vi "Serial Reaction Time Task Controller.vi"() -> ()   [LabVIEW 2016]
uses:
  <vilib>/LabVIEW Interface for Arduino/Type Defs/Board Type.ctl
  <vilib>/Utility/file.llb/Read Delimited Spreadsheet (DBL).vi
  <vilib>/Utility/file.llb/Write Delimited Spreadsheet (DBL).vi
  <vilib>/Utility/file.llb/Write To Spreadsheet File (DBL).vi
  <vilib>/LabVIEW Interface for Arduino/LabVIEW Interface for Arduino.lvlib
panel:
  in  "Debug Mode":bool
  in  "Load Last":bool
  in  "Timeout (sec)":dbl min=0.0 max=1000.0 step=1.0
  in  "Test Mode":bool
  in  "Test Chamber":i32=1 min=1 max=9 step=1
  out "Array":dbl[][](array[numeric])
  in  "Tone":bool
  in  "# of Pellet":i32 max=1000 step=1
  in  "LH (sec)":dbl min=0.0 max=1000.0 step=1.0
  in  "LED On (sec)":dbl min=0.0 max=1000.0 step=1.0
  in  "ITI (sec)":dbl min=0.0 max=1000.0 step=1.0
  in  "# of total Trial":i32 min=0 max=1000 step=1
  in  "Stepper Step":i32 min=0 step=1
  out "ITI":bool
  out "Hole 9":bool
  out "Hole 8":bool
  out "Hole 7":bool
  out "Hole 6":bool
  out "Hole  6":bool
  out "Hole  7":bool
  out "Hole  8":bool
  out "Hole  9":bool
  out "ITI Remaining":dbl format="%<%M:%S>t"
  out "LH Remaining":dbl(slide) scale=0.0..1.0
  out "Experiment Running":bool
  out "Hole 5":bool
  out "Hole 4":bool
  out "Hole 3":bool
  out "Hole 2":bool
  out "Hole 1":bool
  out "Elapsed Time":dbl format="%<%M:%S>t"
  out "Current Trial":dbl
  out "RT (ms)":dbl
  out "Hole  1":bool
  out "Hole  2":bool
  out "Hole  3":bool
  out "Hole  4":bool
  out "Hole  5":bool
  out "Wrong":bool
  out "Correct":bool
  in  "Choice Mode":string(combo)
  out "Detector 2":i32
  out "LED 2":i32
  in  "Set":bool
  in  "Detector Pin":i32=40
  in  "LED Pin":i32=22
  in  "Path":path
  in  "Start":bool
  # "Indicator LED"
  # "Reaction Hole"
  # "to"
  # "to"
  # "# of Trial"
  # "Indicator"
  # "Reaction"
  # "Correct?"
  # "PR?"
  # "# of PMR"
  # "RT(ms)"
  # "Serial Reaction Time Task Controller\nVer 1.0"
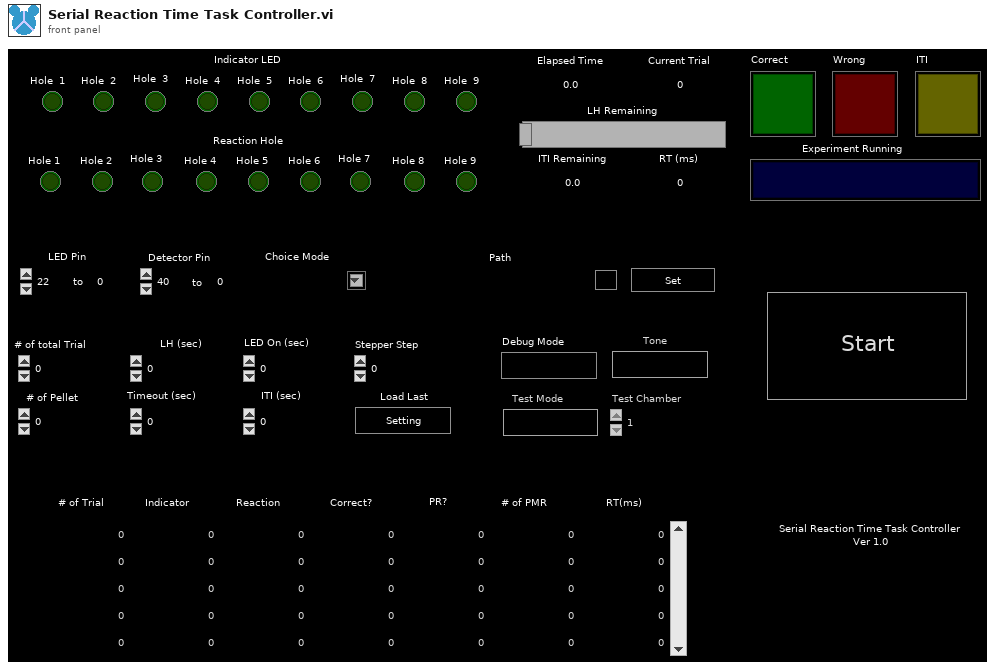
[diagram p1: front panel]
types:
  T1 = typedef "LabVIEW Interface for Arduino.lvlib/Board Type.ctl" = enum16{"Uno", "Dimuelanove w/Atmega 328", "Mega 2560"}
  T2 = enum8{"Enabled", "Disabled", "Disabled and Grayed Out"}
  T3 = typedef "LabVIEW Interface for Arduino.lvlib/Arduino Resource.ctl" = cluster{"VISA resource":refnum<visa-resource-name>, "Board Type":T1, "Connection Type":enum8{"USB / Serial"}, "Bytes Per Packet (15)":u8}
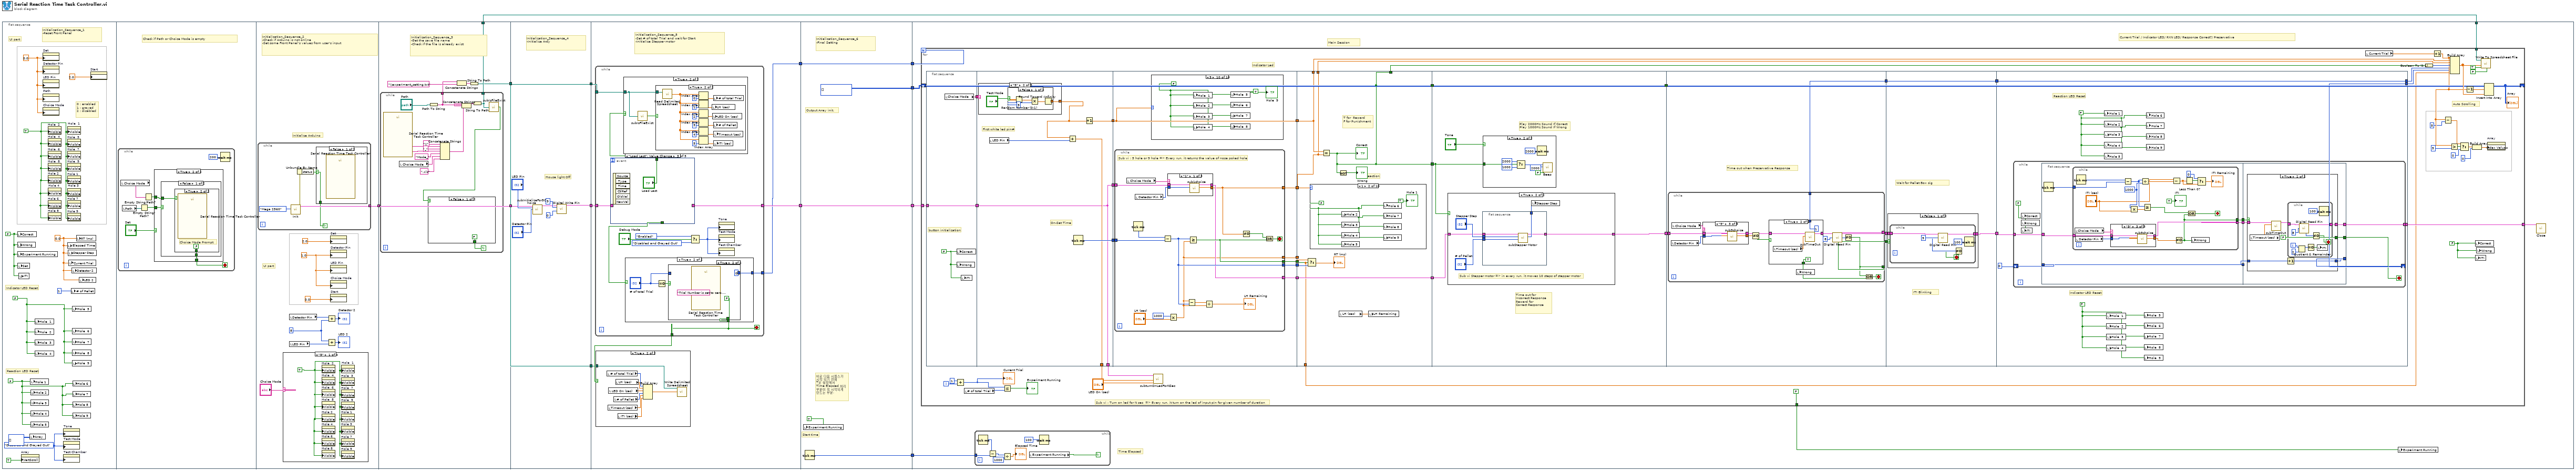
[diagram p0: block diagram]
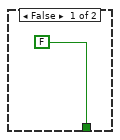
[diagram p2: hidden frame]
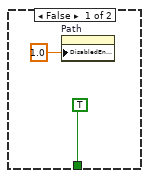
[diagram p3: hidden frame]
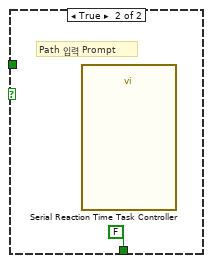
[diagram p4: hidden frame]
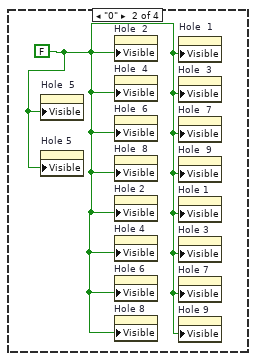
[diagram p5: hidden frame]
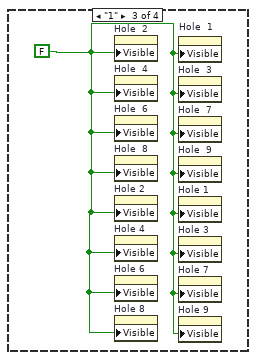
[diagram p6: hidden frame]
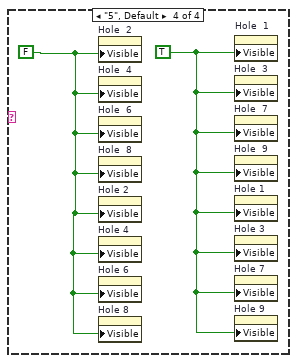
[diagram p7: hidden frame]
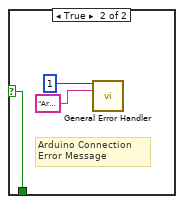
[diagram p8: hidden frame]
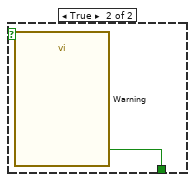
[diagram p9: hidden frame]
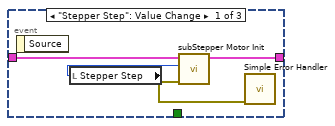
[diagram p11: hidden frame]
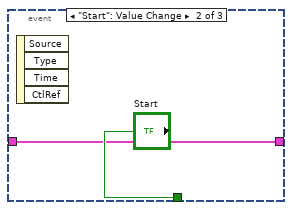
[diagram p12: hidden frame]
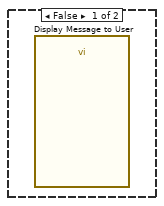
[diagram p14: hidden frame]
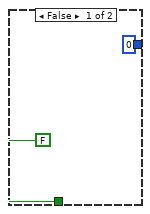
[diagram p15: hidden frame]
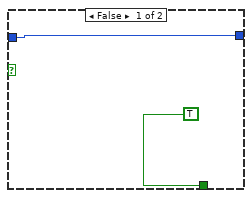
[diagram p16: hidden frame]
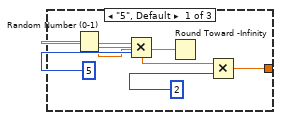
[diagram p17: hidden frame]
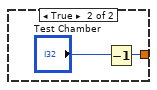
[diagram p18: hidden frame]
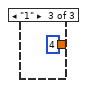
[diagram p19: hidden frame]
diagram:
  n1 = flat-sequence {
    tunnel: [w51] -> w6
    tunnel: [w71] -> w7
    tunnel: w6 -> [w71]
    tunnel: [w70] -> w4
    tunnel: [w67] -> w3
    tunnel: [w88] -> w9
    tunnel: w7 -> [w93]
    tunnel: w3 -> [w92]
    tunnel: [w92] -> w2
    tunnel: [w92] -> w1
    tunnel: [w101] -> w11
    tunnel: [w99] -> w10
    tunnel: w9 -> [w100]
    tunnel: w2 -> [w97]
    tunnel: w1 -> [w96]
    tunnel: [w154] -> w13
    tunnel: [w158] -> w12
    tunnel: w11 -> [w154]
    tunnel: w10 -> [w158]
    tunnel: [w157] -> w8
    tunnel: [i32[][] []] -> w5
    tunnel: w13 -> [w165]
    tunnel: w12 -> [w163]
    tunnel: w8 -> [w162]
    tunnel: w4 -> [w160]
    tunnel: w5 -> [w159]
    frame #0 {
      w14 = T2."Disabled and Grayed Out" ("Disabled")
      w17 = TRUE
      w22 = FALSE
      w23 = FALSE
      w16 = 0.0
      w19 = 0.0
      w18 = FALSE
      # "0 : enabled\n1 : grayed\n2 : disabled"
      # "Initialization_Sequence_1\n-Reset Front Panel"
      # "UI part"
      # "Reaction LED Reset"
      # "Indicator LED Reset"
      n2 = local write "Correct"(w18) -> ()
      n3 = local write "Wrong"(w18) -> ()
      n4 = local write "Experiment Running"(w18) -> ()
      n5 = local write "Set"(w18) -> ()
      n6 = local write "ITI"(w18) -> ()
      n7 = property on="Array" class="Arr (strict)"("VertScroll"=TRUE) -> ()  [unwired: 2 in, 2 out]
      n8 = local write "Array"(i32[][] []) -> ()
      n9 = local write "Hole 1"(w22) -> ()
      n10 = local write "Hole 2"(w22) -> ()
      n11 = local write "Hole 3"(w22) -> ()
      n12 = local write "Hole 4"(w22) -> ()
      n13 = local write "Hole 5"(w22) -> ()
      n14 = local write "Hole  1"(w23) -> ()
      n15 = local write "Hole  2"(w23) -> ()
      n16 = local write "Hole  3"(w23) -> ()
      n17 = local write "Hole  4"(w23) -> ()
      n18 = property on="Set" class="Bool (strict)"("DisabledEnum"=w16) -> ()  [unwired: 2 in, 2 out]
      n19 = property on="Detector Pin" class="DigNum (strict)"("DisabledEnum"=w16) -> ()  [unwired: 2 in, 2 out]
      n20 = property on="LED Pin" class="DigNum (strict)"("DisabledEnum"=w16) -> ()  [unwired: 2 in, 2 out]
      n21 = property on="Path" class="Path"("DisabledEnum"=w16) -> ()  [unwired: 2 in, 2 out]
      n22 = property on="Choice Mode" class="CmbBox"("DisabledEnum"=w16) -> ()  [unwired: 2 in, 2 out]
      n23 = property on="Hole  2" class="Bool (strict)"("Visible"=w17) -> ()  [unwired: 2 in, 2 out]
      n24 = property on="Hole  4" class="Bool (strict)"("Visible"=w17) -> ()  [unwired: 2 in, 2 out]
      n25 = property on="Hole  6" class="Bool (strict)"("Visible"=w17) -> ()  [unwired: 2 in, 2 out]
      n26 = property on="Hole  8" class="Bool (strict)"("Visible"=w17) -> ()  [unwired: 2 in, 2 out]
      n27 = property on="Hole 2" class="Bool (strict)"("Visible"=w17) -> ()  [unwired: 2 in, 2 out]
      n28 = property on="Hole 4" class="Bool (strict)"("Visible"=w17) -> ()  [unwired: 2 in, 2 out]
      n29 = property on="Hole 6" class="Bool (strict)"("Visible"=w17) -> ()  [unwired: 2 in, 2 out]
      n30 = property on="Hole 8" class="Bool (strict)"("Visible"=w17) -> ()  [unwired: 2 in, 2 out]
      n31 = property on="Tone" class="Bool (strict)"("DisabledEnum"=w14) -> ()  [unwired: 2 in, 2 out]
      n32 = property on="Test Mode" class="Bool (strict)"("DisabledEnum"=w14) -> ()  [unwired: 2 in, 2 out]
      n33 = property on="Test Chamber" class="DigNum (strict)"("DisabledEnum"=w14) -> ()  [unwired: 2 in, 2 out]
      n34 = local write "Elapsed Time"(w19) -> ()
      n35 = property on="Hole  1" class="Bool (strict)"("Visible"=w17) -> ()  [unwired: 2 in, 2 out]
      n36 = property on="Hole  3" class="Bool (strict)"("Visible"=w17) -> ()  [unwired: 2 in, 2 out]
      n37 = property on="Hole  7" class="Bool (strict)"("Visible"=w17) -> ()  [unwired: 2 in, 2 out]
      n38 = property on="Hole  9" class="Bool (strict)"("Visible"=w17) -> ()  [unwired: 2 in, 2 out]
      n39 = property on="Hole 1" class="Bool (strict)"("Visible"=w17) -> ()  [unwired: 2 in, 2 out]
      n40 = property on="Hole 3" class="Bool (strict)"("Visible"=w17) -> ()  [unwired: 2 in, 2 out]
      n41 = property on="Hole 7" class="Bool (strict)"("Visible"=w17) -> ()  [unwired: 2 in, 2 out]
      n42 = property on="Hole 9" class="Bool (strict)"("Visible"=w17) -> ()  [unwired: 2 in, 2 out]
      n43 = local write "Stepper Step"(w19) -> ()
      n44 = local write "Current Trial"(w19) -> ()
      n45 = local write "# of Pellet"(1) -> ()
      n46 = local write "Detector 2"(w19) -> ()
      n47 = local write "Hole  5"(w23) -> ()
      n48 = local write "Hole  6"(w23) -> ()
      n49 = local write "Hole  7"(w23) -> ()
      n50 = local write "Hole  8"(w23) -> ()
      n51 = local write "Hole  9"(w23) -> ()
      n52 = local write "Hole 6"(w22) -> ()
      n53 = local write "Hole 7"(w22) -> ()
      n54 = local write "Hole 8"(w22) -> ()
      n55 = local write "Hole 9"(w22) -> ()
      n56 = local write "RT (ms)"(w19) -> ()
      n57 = local write "LED 2"(w19) -> ()
      n58 = property on="Start" class="Bool (strict)"("DisabledEnum"=2.0) -> ()  [unwired: 2 in, 2 out]
    }
    frame #1 {
      # "Check if Path or Choice Mode is empty"
      n59 = while {
        stop <- w31 stop-if-true
        n60 = local read "Choice Mode"() -> (w26:string)
        n61 = local read "Path"() -> (w29:path)
        n62 = Empty String/Path?(string/path=w29) -> (empty?=w30:bool)
        n63 = Empty String/Path?(string/path=w26) -> (empty?=w27:bool)
        n64 = case shown="True" "Set" {
          tunnel: [FALSE w35] -> w31
          tunnel: w30 -> [_ w34]
          tunnel: w27 -> [_ w33]
          frame False {
          }
          frame True {
            n65 = case shown="False" w34 {
              tunnel: [w36 FALSE] -> w35
              tunnel: w33 -> [w37 _]
              frame False {
                n66 = case shown="True" w37 {
                  tunnel: [TRUE FALSE] -> w36
                  frame False {
                    n67 = property on="Path" class="Path"("DisabledEnum"=1.0) -> ()  [unwired: 2 in, 2 out]
                  }
                  frame True {
                    # "Choice Mode Prompt"
                    n68 = call "Serial Reaction Time Task Controller"() -> ()  [unwired: 10 in, 2 out]
                  }
                }
              }
              frame True {
                # "Path 입력 Prompt"
                n69 = call "Serial Reaction Time Task Controller"() -> ()  [unwired: 10 in, 2 out]
              }
            }
          }
        }
        n70 = Wait (ms)(milliseconds to wait=u32 200) -> ()  [unwired: 1 out]
      }
    }
    frame #2 {
      w46 = 8
      w47 = 1.0
      # "Initialize Arduino"
      # "UI part"
      # "Initialization_Sequence_2\n-Check if Arduino is not online\n-Set some Front Panel's values from user's input"
      n71 = while {
        tunnel: [w60] -> w51
        stop <- w57 continue-if-true
        n72 = call <vilib>:"Init.vi"("Board Type (Uno)"=Board_Type."Mega 2560") -> ("Arduino Resource"=w60:T3, "error out"=w59:errorcluster)  [unwired: 17 in]
        n73 = Unbundle By Name(w59) -> ("status"=w58:bool)
        n74 = case shown="False" w58 {
          selector: w58 -> [w62 w63]
          tunnel: [w62 w63] -> w57
          frame False {
            n75 = call "Serial Reaction TIme Task Controller"() -> ()  [unwired: 10 in, 2 out]
          }
          frame True {
            # "Arduino Connection\nError Message"
            n76 = call <vilib>:"General Error Handler.vi"("[error code] (0)"=1, "[error source] (\" \")"="Arduino Connection Error. Check USB port or plug USB port out and in again." ("[error source] (\" \")")) -> ()  [unwired: 9 in, 5 out]
          }
        }
      }
      n77 = case shown="\"9\"" "Choice Mode" {
        frame "9" {
          w52 = TRUE
          n78 = property on="Hole  2" class="Bool (strict)"("Visible"=w52) -> ()  [unwired: 2 in, 2 out]
          n79 = property on="Hole  4" class="Bool (strict)"("Visible"=w52) -> ()  [unwired: 2 in, 2 out]
          n80 = property on="Hole  6" class="Bool (strict)"("Visible"=w52) -> ()  [unwired: 2 in, 2 out]
          n81 = property on="Hole  8" class="Bool (strict)"("Visible"=w52) -> ()  [unwired: 2 in, 2 out]
          n82 = property on="Hole 2" class="Bool (strict)"("Visible"=w52) -> ()  [unwired: 2 in, 2 out]
          n83 = property on="Hole 4" class="Bool (strict)"("Visible"=w52) -> ()  [unwired: 2 in, 2 out]
          n84 = property on="Hole 6" class="Bool (strict)"("Visible"=w52) -> ()  [unwired: 2 in, 2 out]
          n85 = property on="Hole 8" class="Bool (strict)"("Visible"=w52) -> ()  [unwired: 2 in, 2 out]
          n86 = property on="Hole  1" class="Bool (strict)"("Visible"=w52) -> ()  [unwired: 2 in, 2 out]
          n87 = property on="Hole  3" class="Bool (strict)"("Visible"=w52) -> ()  [unwired: 2 in, 2 out]
          n88 = property on="Hole  7" class="Bool (strict)"("Visible"=w52) -> ()  [unwired: 2 in, 2 out]
          n89 = property on="Hole  9" class="Bool (strict)"("Visible"=w52) -> ()  [unwired: 2 in, 2 out]
          n90 = property on="Hole 1" class="Bool (strict)"("Visible"=w52) -> ()  [unwired: 2 in, 2 out]
          n91 = property on="Hole 3" class="Bool (strict)"("Visible"=w52) -> ()  [unwired: 2 in, 2 out]
          n92 = property on="Hole 7" class="Bool (strict)"("Visible"=w52) -> ()  [unwired: 2 in, 2 out]
          n93 = property on="Hole 9" class="Bool (strict)"("Visible"=w52) -> ()  [unwired: 2 in, 2 out]
        }
        frame "0" {
          w53 = FALSE
          n94 = property on="Hole  5" class="Bool (strict)"("Visible"=w53) -> ()  [unwired: 2 in, 2 out]
          n95 = property on="Hole 5" class="Bool (strict)"("Visible"=w53) -> ()  [unwired: 2 in, 2 out]
          n96 = property on="Hole  2" class="Bool (strict)"("Visible"=w53) -> ()  [unwired: 2 in, 2 out]
          n97 = property on="Hole  4" class="Bool (strict)"("Visible"=w53) -> ()  [unwired: 2 in, 2 out]
          n98 = property on="Hole  6" class="Bool (strict)"("Visible"=w53) -> ()  [unwired: 2 in, 2 out]
          n99 = property on="Hole  8" class="Bool (strict)"("Visible"=w53) -> ()  [unwired: 2 in, 2 out]
          n100 = property on="Hole 2" class="Bool (strict)"("Visible"=w53) -> ()  [unwired: 2 in, 2 out]
          n101 = property on="Hole 4" class="Bool (strict)"("Visible"=w53) -> ()  [unwired: 2 in, 2 out]
          n102 = property on="Hole 6" class="Bool (strict)"("Visible"=w53) -> ()  [unwired: 2 in, 2 out]
          n103 = property on="Hole 8" class="Bool (strict)"("Visible"=w53) -> ()  [unwired: 2 in, 2 out]
          n104 = property on="Hole  1" class="Bool (strict)"("Visible"=w53) -> ()  [unwired: 2 in, 2 out]
          n105 = property on="Hole  3" class="Bool (strict)"("Visible"=w53) -> ()  [unwired: 2 in, 2 out]
          n106 = property on="Hole  7" class="Bool (strict)"("Visible"=w53) -> ()  [unwired: 2 in, 2 out]
          n107 = property on="Hole  9" class="Bool (strict)"("Visible"=w53) -> ()  [unwired: 2 in, 2 out]
          n108 = property on="Hole 1" class="Bool (strict)"("Visible"=w53) -> ()  [unwired: 2 in, 2 out]
          n109 = property on="Hole 3" class="Bool (strict)"("Visible"=w53) -> ()  [unwired: 2 in, 2 out]
          n110 = property on="Hole 7" class="Bool (strict)"("Visible"=w53) -> ()  [unwired: 2 in, 2 out]
          n111 = property on="Hole 9" class="Bool (strict)"("Visible"=w53) -> ()  [unwired: 2 in, 2 out]
        }
        frame "1" {
          w54 = FALSE
          n112 = property on="Hole  2" class="Bool (strict)"("Visible"=w54) -> ()  [unwired: 2 in, 2 out]
          n113 = property on="Hole  4" class="Bool (strict)"("Visible"=w54) -> ()  [unwired: 2 in, 2 out]
          n114 = property on="Hole  6" class="Bool (strict)"("Visible"=w54) -> ()  [unwired: 2 in, 2 out]
          n115 = property on="Hole  8" class="Bool (strict)"("Visible"=w54) -> ()  [unwired: 2 in, 2 out]
          n116 = property on="Hole 2" class="Bool (strict)"("Visible"=w54) -> ()  [unwired: 2 in, 2 out]
          n117 = property on="Hole 4" class="Bool (strict)"("Visible"=w54) -> ()  [unwired: 2 in, 2 out]
          n118 = property on="Hole 6" class="Bool (strict)"("Visible"=w54) -> ()  [unwired: 2 in, 2 out]
          n119 = property on="Hole 8" class="Bool (strict)"("Visible"=w54) -> ()  [unwired: 2 in, 2 out]
          n120 = property on="Hole  1" class="Bool (strict)"("Visible"=w54) -> ()  [unwired: 2 in, 2 out]
          n121 = property on="Hole  3" class="Bool (strict)"("Visible"=w54) -> ()  [unwired: 2 in, 2 out]
          n122 = property on="Hole  7" class="Bool (strict)"("Visible"=w54) -> ()  [unwired: 2 in, 2 out]
          n123 = property on="Hole  9" class="Bool (strict)"("Visible"=w54) -> ()  [unwired: 2 in, 2 out]
          n124 = property on="Hole 1" class="Bool (strict)"("Visible"=w54) -> ()  [unwired: 2 in, 2 out]
          n125 = property on="Hole 3" class="Bool (strict)"("Visible"=w54) -> ()  [unwired: 2 in, 2 out]
          n126 = property on="Hole 7" class="Bool (strict)"("Visible"=w54) -> ()  [unwired: 2 in, 2 out]
          n127 = property on="Hole 9" class="Bool (strict)"("Visible"=w54) -> ()  [unwired: 2 in, 2 out]
        }
        frame "5", Default {
          w55 = TRUE
          w56 = FALSE
          n128 = property on="Hole  2" class="Bool (strict)"("Visible"=w56) -> ()  [unwired: 2 in, 2 out]
          n129 = property on="Hole  4" class="Bool (strict)"("Visible"=w56) -> ()  [unwired: 2 in, 2 out]
          n130 = property on="Hole  6" class="Bool (strict)"("Visible"=w56) -> ()  [unwired: 2 in, 2 out]
          n131 = property on="Hole  8" class="Bool (strict)"("Visible"=w56) -> ()  [unwired: 2 in, 2 out]
          n132 = property on="Hole 2" class="Bool (strict)"("Visible"=w56) -> ()  [unwired: 2 in, 2 out]
          n133 = property on="Hole 4" class="Bool (strict)"("Visible"=w56) -> ()  [unwired: 2 in, 2 out]
          n134 = property on="Hole 6" class="Bool (strict)"("Visible"=w56) -> ()  [unwired: 2 in, 2 out]
          n135 = property on="Hole 8" class="Bool (strict)"("Visible"=w56) -> ()  [unwired: 2 in, 2 out]
          n136 = property on="Hole  1" class="Bool (strict)"("Visible"=w55) -> ()  [unwired: 2 in, 2 out]
          n137 = property on="Hole  3" class="Bool (strict)"("Visible"=w55) -> ()  [unwired: 2 in, 2 out]
          n138 = property on="Hole  7" class="Bool (strict)"("Visible"=w55) -> ()  [unwired: 2 in, 2 out]
          n139 = property on="Hole  9" class="Bool (strict)"("Visible"=w55) -> ()  [unwired: 2 in, 2 out]
          n140 = property on="Hole 1" class="Bool (strict)"("Visible"=w55) -> ()  [unwired: 2 in, 2 out]
          n141 = property on="Hole 3" class="Bool (strict)"("Visible"=w55) -> ()  [unwired: 2 in, 2 out]
          n142 = property on="Hole 7" class="Bool (strict)"("Visible"=w55) -> ()  [unwired: 2 in, 2 out]
          n143 = property on="Hole 9" class="Bool (strict)"("Visible"=w55) -> ()  [unwired: 2 in, 2 out]
        }
      }
      n144 = local read "Detector Pin"() -> (w45:i32)
      n145 = local read "LED Pin"() -> (w43:i32)
      n146 = Add(x=w45, y=w46) -> (x+y=→"Detector 2":i32)
      n147 = Add(x=w46, y=w43) -> (x+y=→"LED 2":i32)
      n148 = property on="Set" class="Bool (strict)"("DisabledEnum"=2.0) -> ()  [unwired: 2 in, 2 out]
      n149 = property on="Detector Pin" class="DigNum (strict)"("DisabledEnum"=w47) -> ()  [unwired: 2 in, 2 out]
      n150 = property on="LED Pin" class="DigNum (strict)"("DisabledEnum"=w47) -> ()  [unwired: 2 in, 2 out]
      n151 = property on="Choice Mode" class="CmbBox"("DisabledEnum"=w47) -> ()  [unwired: 2 in, 2 out]
      n152 = property on="Start" class="Bool (strict)"("DisabledEnum"=0.0) -> ()  [unwired: 2 in, 2 out]
    }
    frame #3 {
      # "Initialization_Sequence_3\n-Get the save file name\n-Check if the file is already exist"
      n153 = while {
        tunnel: [w77] -> w70
        tunnel: [w75] -> w66
        stop <- w78 continue-if-true
        n154 = call "Serial Reaction Time Task Controller"() -> ("Subject number"=w84:string, "Experiment name"=w82:string)  [unwired: 16 in, 2 out]
        n155 = local read "Choice Mode"() -> (w72:string)
        n156 = Path To String(path="Path") -> (string=w75:string)
        n157 = Concatenate Strings("\\", w82, "_", w84, "Mode_", w72, ".xls") -> (w80:string)
        n158 = Concatenate Strings(w75, w80) -> (w81:string)
        n159 = String To Path(string=w81) -> (path=w77:path)
        n160 = call "subIsFileExist.vi"("Path"=w77) -> ("isFileExist"=w79:bool)
        n161 = case shown="False" w79 {
          tunnel: [FALSE w87] -> w78
          frame False {
          }
          frame True {
            n162 = call "Warning"() -> ("Change"=w87:bool)  [unwired: 18 in, 1 out]
          }
        }
      }
      n163 = Concatenate Strings(w66, "\\experiment_setting.txt" ("string")) -> (w68:string)
      n164 = String To Path(string=w68) -> (path=w67:path)
    }
    frame #4 {
      # "House light Off"
      # "Initialization_Sequence_4\n-Initialize Ardy"
      n165 = call "subInitializeFor5Choice.vi"("Arduino Resource"=w93, "LED Start Pin"="LED Pin", "Detector Start Pin"="Detector Pin") -> ("Arduino Resource 2"=w89:T3)  [unwired: 11 in, 1 out]
      n166 = call <vilib>:"Digital Write Pin.vi"("Arduino Resource"=w89, "Digital I/O Pin (0)"=9, "Value (0)"=0) -> ("Arduino Resource"=w88:T3)  [unwired: 11 in, 1 out]
    }
    frame #5 {
      # "Initialization_Sequence_5\n-Set # of total Trial and wait for Start\n-Initialize Stepper motor"
      n167 = while {
        tunnel: [w112] -> w101
        tunnel: w100 -> [w113]
        tunnel: [w120] -> w99
        tunnel: [w115] -> w98
        tunnel: w96 -> [w114]
        stop <- w115 stop-if-true
        n168 = event shown="[2] \"Load Last\": Value Change" {
          selector: _ -> [_ _ _]
          dyn-events: _ -> [_ _ _]
          timeout: _ -> [_ _ _]
          tunnel: w113 -> [w124 w125 _]
          tunnel: [w123 w125 _] -> w112
          tunnel: [_ "Start" _] -> w111
          tunnel: [_ _ "Load Last"] -> w110
          event "Stepper Step": Value Change {
            n169 = event-data() -> ()  [unwired: 1 in, 1 out]
            n170 = local read "Stepper Step"() -> (w121:i32)
            n171 = call "subStepper Motor Init.vi"("Numeric"=w121, "Arduino Resource"=w124) -> ("error out"=w122:errorcluster, "Arduino Resource 2"=w123:T3)  [unwired: 8 in]
            n172 = call <vilib>:"Simple Error Handler.vi"("error in (no error)"=w122) -> ()  [unwired: 4 in, 5 out]
          }
          event "Start": Value Change {
            n173 = event-data() -> ()  [unwired: 1 in, 4 out]
          }
          event "Load Last": Value Change {
            n174 = event-data() -> ()  [unwired: 1 in, 6 out]
          }
        }
        n175 = case shown="True" w110 {
          tunnel: w114 -> [_ w129]
          frame False {
          }
          frame True {
            n176 = call "subIsFileExist.vi"("Path"=w129) -> ("isFileExist"=w128:bool)
            n177 = case shown="True" w128 {
              tunnel: w129 -> [_ w131]
              frame False {
                n178 = call "Display Message to User"() -> ()  [unwired: 10 in, 2 out]
              }
              frame True {
                n179 = call-poly <vilib>:"Read Delimited Spreadsheet.vi"("file path (dialog if empty)"=w131) -> ("first row"=w130:dbl[])  [unwired: 9 in, 5 out]
                n180 = Index Array(array=w130, index=0) -> (element=w143:dbl)
                n181 = Index Array(array=w130, index=1) -> (element=w142:dbl)
                n182 = Index Array(array=w130, index=2) -> (element=w141:dbl)
                n183 = Index Array(array=w130, index=3) -> (element=w140:dbl)
                n184 = Index Array(array=w130, index=4) -> (element=w139:dbl)
                n185 = Index Array(array=w130, index=5) -> (element=w138:dbl)
                n186 = local write "LH (sec)"(w142) -> ()
                n187 = local write "LED On (sec)"(w141) -> ()
                n188 = local write "# of total Trial"(w143) -> ()
                n189 = local write "# of Pellet"(w140) -> ()
                n190 = local write "Timeout (sec)"(w139) -> ()
                n191 = local write "ITI (sec)"(w138) -> ()
              }
            }
          }
        }
        n192 = case shown="True" w111 {
          tunnel: [0 ("# of total Trial") w146] -> w120
          tunnel: [FALSE w148] -> w115
          frame False {
          }
          frame True {
            n193 = Equal To 0?(x="# of total Trial") -> (x = 0?=w149:bool)
            n194 = case shown="True" w149 {
              tunnel: [TRUE FALSE] -> w148
              tunnel: "# of total Trial" -> [w151 _]
              tunnel: [w151 0 ("# of total Trial")] -> w146
              frame False {
              }
              frame True {
                (unwired) "Trial Number is set to zero. Please change the value" ("error source (\" \")")
                n195 = call "Serial Reaction Time Task Controller"() -> ()  [unwired: 10 in, 2 out]
              }
            }
          }
        }
        n196 = Select(t=T2."Enabled" ("Disabled"), s="Debug Mode", f=T2."Disabled and Grayed Out" ("Disabled")) -> (s? t:f=w116:T2)
        n197 = property on="Tone" class="Bool (strict)"("DisabledEnum"=w116) -> ()  [unwired: 2 in, 2 out]
        n198 = property on="Test Mode" class="Bool (strict)"("DisabledEnum"=w116) -> ()  [unwired: 2 in, 2 out]
        n199 = property on="Test Chamber" class="DigNum (strict)"("DisabledEnum"=w116) -> ()  [unwired: 2 in, 2 out]
      }
      n200 = case shown="True" w98 {
        tunnel: w97 -> [_ w103]
        frame False {
        }
        frame True {
          n201 = local read "# of total Trial"() -> (w109:i32)
          n202 = local read "Timeout (sec)"() -> (w105:dbl)
          n203 = local read "LED On (sec)"() -> (w107:dbl)
          n204 = local read "# of Pellet"() -> (w106:i32)
          n205 = local read "LH (sec)"() -> (w108:dbl)
          n206 = local read "ITI (sec)"() -> (w104:dbl)
          n207 = Build Array(w109, w108, w107, w106, w105, w104) -> (w102:dbl[])
          n208 = call-poly <vilib>:"Write Delimited Spreadsheet.vi"("file path (dialog if empty)"=w103, "1D data"=w102) -> ()  [unwired: 12 in, 2 out]
        }
      }
    }
    frame #6 {
      # "Output Array init."
      # "Initialization_Sequence_6\n-Final Setting"
      # "바로 다음 시퀀스가\n시작 되기 전에 \nT로 설정해서 \nTime Elapsed 처리\n부분이 꼭 시작되게\n만드는 부분."
      # "Start time"
      n209 = local write "Experiment Running"(TRUE) -> ()
      n210 = Tick Count (ms)() -> (millisecond timer value=w157:u32)
    }
    frame #7 {
      # "Current Trial / Indicator LED/ RXN LED/ Response Correct?/ Preservative"
      # "Time Elapsed"
      # "Main Session"
      n211 = for {
        N: w163 -> [_]
        tunnel: w165 -> [w224]
        tunnel: [w220] -> w164
        tunnel: [FALSE] -> w161
        tunnel: w160 -> [w207]
        shift-right: [w200] -> _
        shift-left: w159 -> [w201]
        i -> [w217]
        w174 = FALSE
        # "Indicator Led"
        # "Auto Scrolling"
        # "Sub vi : Turn on led for N sec  => Every run, it turn on the led of input pin for given number of duration"
        n212 = flat-sequence {
          tunnel: w224 -> [w232]
          tunnel: [w232] -> w223
          tunnel: [w231] -> w208
          tunnel: [w233] -> w229
          tunnel: [w239] -> w228
          tunnel: w223 -> [w237]
          tunnel: [w237] -> w212
          tunnel: [w238] -> w213
          tunnel: [w237] -> w222
          tunnel: w208 -> [w235]
          tunnel: w229 -> [w256]
          tunnel: w228 -> [w262]
          tunnel: [w256] -> w227
          tunnel: [w261] -> w226
          tunnel: [w260] -> w225
          tunnel: w222 -> [w259]
          tunnel: [w258] -> w221
          tunnel: [w257] -> w219
          tunnel: [w255] -> w209
          tunnel: w227 -> [w314]
          tunnel: w226 -> [w309]
          tunnel: w225 -> [w316]
          tunnel: [w318] -> w185
          tunnel: w221 -> [w318]
          tunnel: [w312] -> w184
          tunnel: w219 -> [w315]
          tunnel: [w314] -> w206
          tunnel: [w309] -> w205
          tunnel: [w312] -> w218
          tunnel: w209 -> [w313]
          tunnel: [w312] -> w183
          tunnel: [w311] -> w175
          tunnel: [w341] -> w187
          tunnel: [w340] -> w186
          tunnel: w183 -> [w340]
          tunnel: w184 -> [w338]
          tunnel: w185 -> [w342]
          tunnel: w187 -> [w366]
          tunnel: [w365] -> w181
          tunnel: w186 -> [_]
          tunnel: [w364] -> w179
          tunnel: [w363] -> w177
          tunnel: w181 -> [w403]
          tunnel: [w402] -> w180
          tunnel: w179 -> [w404]
          tunnel: [w404] -> w178
          tunnel: w177 -> [w401]
          tunnel: w180 -> [w417]
          tunnel: [w418] -> w220
          tunnel: w178 -> [w416]
          tunnel: [w416] -> w182
          tunnel: [w414] -> w176
          frame #0 {
            w230 = FALSE
            # "button initialization"
            n213 = local read "Choice Mode"() -> (w231:string)
            n214 = local write "Correct"(w230) -> ()
            n215 = local write "Wrong"(w230) -> ()
            n216 = local write "ITI"(w230) -> ()
          }
          frame #1 {
            # "On-Set Time"
            # "First white led pin#"
            n217 = case shown="\"9\"" w235 {
              tunnel: [w240 w247 4] -> w234
              frame "5", Default {
                n218 = Random Number (0-1)() -> (number: 0 to 1=w244:dbl)
                n219 = Multiply(x=w244, y=5) -> (x*y=w241:dbl)
                n220 = Round Toward -Infinity(1:w241) -> (0:w242:dbl)
                n221 = Multiply(x=w242, y=2) -> (x*y=w240:dbl)
              }
              frame "9" {
                n222 = case shown="False" "Test Mode" {
                  tunnel: [w248 w252] -> w247
                  frame False {
                    n223 = Random Number (0-1)() -> (number: 0 to 1=w251:dbl)
                    n224 = Multiply(x=w251, y=9) -> (x*y=w249:dbl)
                    n225 = Round Toward -Infinity(1:w249) -> (0:w248:dbl)
                  }
                  frame True {
                    n226 = Decrement(x="Test Chamber") -> (x-1=w252:i32)
                  }
                }
              }
              frame "1" {
              }
            }
            n227 = local read "LED Pin"() -> (w236:i32)
            n228 = Add(x=w234, y=w236) -> (x+y=w238:dbl)
            n229 = Tick Count (ms)() -> (millisecond timer value=w239:u32)
            n230 = Increment(x=w234) -> (x+1=w233:dbl)
          }
          frame #2 {
            n231 = while {
              tunnel: w262 -> [w294]
              tunnel: [w287] -> w261
              tunnel: [w291] -> w260
              tunnel: w259 -> [w289]
              tunnel: [w288] -> w258
              tunnel: [w292] -> w257
              tunnel: [w283] -> w255
              stop <- w296 stop-if-true
              # "Sub vi : 5 hole or 9 hole => Every run, it returns the value of nose poked hole"
              n232 = local read "Choice Mode"() -> (w290:string)
              n233 = Tick Count (ms)() -> (millisecond timer value=w293:u32)
              n234 = local read "Detector Pin"() -> (w284:i32)
              n235 = Subtract(x=w293, y=w294) -> (x-y=w291:u32)
              n236 = case shown="\"1\"" w290 {
                tunnel: [w299 w303 w308] -> w288
                tunnel: w289 -> [w300 w304 w306]
                tunnel: [w298 w302 w307] -> w287
                tunnel: w284 -> [w297 w301 w305]
                frame "1" {
                  n237 = call "sub1choice.vi"("Detector Start Pin"=w297, "Arduino Resource"=w300) -> ("Numeric"=w298:dbl, "Arduino Resource 2"=w299:T3)  [unwired: 7 in, 1 out]
                }
                frame "5", Default {
                  n238 = call "sub5choice.vi"("Detector Start Pin"=w301, "Arduino Resource"=w304) -> ("Numeric"=w302:dbl, "Arduino Resource 2"=w303:T3)  [unwired: 7 in, 1 out]
                }
                frame "9" {
                  n239 = call "sub9choice.vi"("Detector Start Pin"=w305, "Arduino Resource"=w306) -> ("Ouput"=w307:dbl, "Arduino Resource 2"=w308:T3)  [unwired: 7 in, 1 out]
                }
              }
              n240 = Multiply(x=1000, y="LH (sec)") -> (x*y=w283:dbl)
              n241 = Subtract(x=w283, y=w291) -> (x-y=w282:dbl)
              n242 = Greater Or Equal?(x=w291, y=w283) -> (x >= y?=w292:bool)
              n243 = Divide(x=w282, y=w283) -> (x/y=→"LH Remaining":dbl)
              n244 = Not Equal To 0?(x=w287) -> (x != 0?=w295:bool)
              n245 = Or(x=w295, y=w292) -> (x .or. y?=w296:bool)
            }
            n246 = case shown="9" w256 {
              frame 0, Default {
              }
              frame 1 {
                w263 = FALSE
                n247 = local write "Hole  2"(w263) -> ()
                n248 = local write "Hole  3"(w263) -> ()
                n249 = local write "Hole  4"(w263) -> ()
                n250 = local write "Hole  5"(w263) -> ()
                n251 = local write "Hole  6"(w263) -> ()
                n252 = local write "Hole  7"(w263) -> ()
                n253 = local write "Hole  8"(w263) -> ()
                n254 = local write "Hole  9"(w263) -> ()
                "Hole  1" <- TRUE
              }
              frame 2 {
                w265 = FALSE
                n255 = local write "Hole  1"(w265) -> ()
                n256 = local write "Hole  3"(w265) -> ()
                n257 = local write "Hole  4"(w265) -> ()
                n258 = local write "Hole  5"(w265) -> ()
                n259 = local write "Hole  6"(w265) -> ()
                n260 = local write "Hole  7"(w265) -> ()
                n261 = local write "Hole  8"(w265) -> ()
                n262 = local write "Hole  9"(w265) -> ()
                "Hole  2" <- TRUE
              }
              frame 3 {
                w267 = FALSE
                n263 = local write "Hole  1"(w267) -> ()
                n264 = local write "Hole  2"(w267) -> ()
                n265 = local write "Hole  4"(w267) -> ()
                n266 = local write "Hole  5"(w267) -> ()
                n267 = local write "Hole  6"(w267) -> ()
                n268 = local write "Hole  7"(w267) -> ()
                n269 = local write "Hole  8"(w267) -> ()
                n270 = local write "Hole  9"(w267) -> ()
                "Hole  3" <- TRUE
              }
              frame 4 {
                w269 = FALSE
                n271 = local write "Hole  1"(w269) -> ()
                n272 = local write "Hole  2"(w269) -> ()
                n273 = local write "Hole  3"(w269) -> ()
                n274 = local write "Hole  5"(w269) -> ()
                n275 = local write "Hole  6"(w269) -> ()
                n276 = local write "Hole  7"(w269) -> ()
                n277 = local write "Hole  8"(w269) -> ()
                n278 = local write "Hole  9"(w269) -> ()
                "Hole  4" <- TRUE
              }
              frame 5 {
                w271 = FALSE
                n279 = local write "Hole  1"(w271) -> ()
                n280 = local write "Hole  2"(w271) -> ()
                n281 = local write "Hole  3"(w271) -> ()
                n282 = local write "Hole  4"(w271) -> ()
                n283 = local write "Hole  6"(w271) -> ()
                n284 = local write "Hole  7"(w271) -> ()
                n285 = local write "Hole  8"(w271) -> ()
                n286 = local write "Hole  9"(w271) -> ()
                "Hole  5" <- TRUE
              }
              frame 6 {
                w274 = FALSE
                n287 = local write "Hole  1"(w274) -> ()
                n288 = local write "Hole  2"(w274) -> ()
                n289 = local write "Hole  3"(w274) -> ()
                n290 = local write "Hole  4"(w274) -> ()
                n291 = local write "Hole  5"(w274) -> ()
                n292 = local write "Hole  7"(w274) -> ()
                n293 = local write "Hole  8"(w274) -> ()
                n294 = local write "Hole  9"(w274) -> ()
                "Hole  6" <- TRUE
              }
              frame 7 {
                w276 = FALSE
                n295 = local write "Hole  1"(w276) -> ()
                n296 = local write "Hole  2"(w276) -> ()
                n297 = local write "Hole  3"(w276) -> ()
                n298 = local write "Hole  4"(w276) -> ()
                n299 = local write "Hole  5"(w276) -> ()
                n300 = local write "Hole  6"(w276) -> ()
                n301 = local write "Hole  8"(w276) -> ()
                n302 = local write "Hole  9"(w276) -> ()
                "Hole  7" <- TRUE
              }
              frame 8 {
                w278 = FALSE
                n303 = local write "Hole  1"(w278) -> ()
                n304 = local write "Hole  2"(w278) -> ()
                n305 = local write "Hole  3"(w278) -> ()
                n306 = local write "Hole  4"(w278) -> ()
                n307 = local write "Hole  5"(w278) -> ()
                n308 = local write "Hole  6"(w278) -> ()
                n309 = local write "Hole  7"(w278) -> ()
                n310 = local write "Hole  9"(w278) -> ()
                "Hole  8" <- TRUE
              }
              frame 9 {
                w280 = FALSE
                n311 = local write "Hole  1"(w280) -> ()
                n312 = local write "Hole  2"(w280) -> ()
                n313 = local write "Hole  3"(w280) -> ()
                n314 = local write "Hole  4"(w280) -> ()
                n315 = local write "Hole  5"(w280) -> ()
                n316 = local write "Hole  6"(w280) -> ()
                n317 = local write "Hole  7"(w280) -> ()
                n318 = local write "Hole  8"(w280) -> ()
                "Hole  9" <- TRUE
              }
            }
          }
          frame #3 {
            # "Reaction"
            # "T for  Reward\nF for Punishment"
            n319 = Select(t=w313, s=w315, f=w316) -> (s? t:f=w311:dbl)
            "RT (ms)" <- w311
            n320 = case shown="1" w309 {
              frame 0, Default {
                w319 = TRUE
                n321 = local write "Hole 1"(w319) -> ()
                n322 = local write "Hole 2"(w319) -> ()
                n323 = local write "Hole 3"(w319) -> ()
                n324 = local write "Hole 4"(w319) -> ()
                n325 = local write "Hole 5"(w319) -> ()
                n326 = local write "Hole 6"(w319) -> ()
                n327 = local write "Hole 7"(w319) -> ()
                n328 = local write "Hole 8"(w319) -> ()
                n329 = local write "Hole 9"(w319) -> ()
              }
              frame 1 {
                w320 = FALSE
                n330 = local write "Hole 2"(w320) -> ()
                n331 = local write "Hole 3"(w320) -> ()
                n332 = local write "Hole 4"(w320) -> ()
                n333 = local write "Hole 5"(w320) -> ()
                n334 = local write "Hole 6"(w320) -> ()
                n335 = local write "Hole 7"(w320) -> ()
                n336 = local write "Hole 8"(w320) -> ()
                n337 = local write "Hole 9"(w320) -> ()
                "Hole 1" <- TRUE
              }
              frame 2 {
                w322 = FALSE
                n338 = local write "Hole 1"(w322) -> ()
                n339 = local write "Hole 3"(w322) -> ()
                n340 = local write "Hole 4"(w322) -> ()
                n341 = local write "Hole 5"(w322) -> ()
                n342 = local write "Hole 6"(w322) -> ()
                n343 = local write "Hole 7"(w322) -> ()
                n344 = local write "Hole 8"(w322) -> ()
                n345 = local write "Hole 9"(w322) -> ()
                "Hole 2" <- TRUE
              }
              frame 3 {
                w324 = FALSE
                n346 = local write "Hole 1"(w324) -> ()
                n347 = local write "Hole 2"(w324) -> ()
                n348 = local write "Hole 4"(w324) -> ()
                n349 = local write "Hole 5"(w324) -> ()
                n350 = local write "Hole 6"(w324) -> ()
                n351 = local write "Hole 7"(w324) -> ()
                n352 = local write "Hole 8"(w324) -> ()
                n353 = local write "Hole 9"(w324) -> ()
                "Hole 3" <- TRUE
              }
              frame 4 {
                w326 = FALSE
                n354 = local write "Hole 1"(w326) -> ()
                n355 = local write "Hole 2"(w326) -> ()
                n356 = local write "Hole 3"(w326) -> ()
                n357 = local write "Hole 5"(w326) -> ()
                n358 = local write "Hole 6"(w326) -> ()
                n359 = local write "Hole 7"(w326) -> ()
                n360 = local write "Hole 8"(w326) -> ()
                n361 = local write "Hole 9"(w326) -> ()
                "Hole 4" <- TRUE
              }
              frame 5 {
                w328 = FALSE
                n362 = local write "Hole 1"(w328) -> ()
                n363 = local write "Hole 2"(w328) -> ()
                n364 = local write "Hole 3"(w328) -> ()
                n365 = local write "Hole 4"(w328) -> ()
                n366 = local write "Hole 6"(w328) -> ()
                n367 = local write "Hole 7"(w328) -> ()
                n368 = local write "Hole 8"(w328) -> ()
                n369 = local write "Hole 9"(w328) -> ()
                "Hole 5" <- TRUE
              }
              frame 6 {
                w331 = FALSE
                n370 = local write "Hole 1"(w331) -> ()
                n371 = local write "Hole 2"(w331) -> ()
                n372 = local write "Hole 3"(w331) -> ()
                n373 = local write "Hole 4"(w331) -> ()
                n374 = local write "Hole 5"(w331) -> ()
                n375 = local write "Hole 7"(w331) -> ()
                n376 = local write "Hole 8"(w331) -> ()
                n377 = local write "Hole 9"(w331) -> ()
                "Hole 6" <- TRUE
              }
              frame 7 {
                w333 = FALSE
                n378 = local write "Hole 1"(w333) -> ()
                n379 = local write "Hole 2"(w333) -> ()
                n380 = local write "Hole 3"(w333) -> ()
                n381 = local write "Hole 4"(w333) -> ()
                n382 = local write "Hole 5"(w333) -> ()
                n383 = local write "Hole 6"(w333) -> ()
                n384 = local write "Hole 8"(w333) -> ()
                n385 = local write "Hole 9"(w333) -> ()
                "Hole 7" <- TRUE
              }
              frame 8 {
                w335 = FALSE
                n386 = local write "Hole 1"(w335) -> ()
                n387 = local write "Hole 2"(w335) -> ()
                n388 = local write "Hole 3"(w335) -> ()
                n389 = local write "Hole 4"(w335) -> ()
                n390 = local write "Hole 5"(w335) -> ()
                n391 = local write "Hole 6"(w335) -> ()
                n392 = local write "Hole 7"(w335) -> ()
                n393 = local write "Hole 9"(w335) -> ()
                "Hole 8" <- TRUE
              }
              frame 9 {
                w337 = FALSE
                n394 = local write "Hole 1"(w337) -> ()
                n395 = local write "Hole 2"(w337) -> ()
                n396 = local write "Hole 3"(w337) -> ()
                n397 = local write "Hole 4"(w337) -> ()
                n398 = local write "Hole 5"(w337) -> ()
                n399 = local write "Hole 6"(w337) -> ()
                n400 = local write "Hole 7"(w337) -> ()
                n401 = local write "Hole 8"(w337) -> ()
                "Hole 9" <- TRUE
              }
            }
            n402 = Equal?(x=w314, y=w309) -> (x = y?=w312:bool)
            "Correct" <- w312
            n403 = Not(x=w312) -> (.not. x?=→"Wrong":bool)
            n404 = local read "LH (sec)"() -> (w310:dbl)
            n405 = local write "LH Remaining"(w310) -> ()
          }
          frame #4 {
            # "Play 2000Hz Sound If Correct\nPlay 1000Hz Sound If Wrong"
            # "Time out for\nIncorrect Response\nReward for\nCorrect Response"
            n406 = case shown="True" w338 {
              tunnel: w342 -> [w351 w355]
              tunnel: [w350 w354] -> w341
              frame False {
                n407 = call "subTimeOut.vi"("Timeout (sec)"="Timeout (sec)", "Arduino Resource"=w351) -> ("Arduino Resource 2"=w350:T3)  [unwired: 9 in]
              }
              frame True {
                # "Sub vi Stepper motor => in every run, it moves 10 steps of stepper motor"
                n408 = flat-sequence {
                  tunnel: "Stepper Step" -> [w361]
                  tunnel: [w362] -> w356
                  tunnel: w355 -> [w360]
                  tunnel: [w359] -> w354
                  tunnel: "# of Pellet" -> [w358]
                  frame #0 {
                    n409 = call "subStepper Motor.vi"("# of Pellet"=w358, "Numeric"=w361, "Arduino Resource"=w360) -> ("Stepper Step"=w362:i32, "Arduino Resource 2"=w359:T3)  [unwired: 6 in, 1 out]
                  }
                }
                n410 = local write "Stepper Step"(w356) -> ()
              }
            }
            n411 = case shown="True" "Tone" {
              tunnel: w338 -> [_ w349]
              frame False {
              }
              frame True {
                n412 = Select(t=u32 2000, s=w349, f=u32 1000) -> (s? t:f=w345:u32)
                n413 = Wait (ms)(milliseconds to wait=u32 2000) -> ()  [unwired: 1 out]
                n414 = call <vilib>:"Beep.vi"("use system alert? (T)"=FALSE, "duration (msec)"=u32 2000, "frequency (Hz)"=w345) -> ()  [unwired: 9 in]
              }
            }
          }
          frame #5 {
            # "Time out when Preservative Response"
            n415 = while {
              tunnel: w366 -> [w374]
              tunnel: [w380] -> w365
              tunnel: [w370] -> w364
              tunnel: [w368] -> w363
              stop <- w369 stop-if-true
              n416 = local read "Detector Pin"() -> (w377:i32)
              n417 = local read "Choice Mode"() -> (w376:string)
              n418 = case shown="\"9\"" w376 {
                tunnel: [w391 w395 w400] -> w372
                tunnel: w374 -> [w392 w396 w398]
                tunnel: [w390 w394 w399] -> w375
                tunnel: w377 -> [w389 w393 w397]
                frame "1" {
                  n419 = call "sub1choice.vi"("Detector Start Pin"=w389, "Arduino Resource"=w392) -> ("Numeric"=w390:dbl, "Arduino Resource 2"=w391:T3)  [unwired: 7 in, 1 out]
                }
                frame "5", Default {
                  n420 = call "sub5choice.vi"("Detector Start Pin"=w393, "Arduino Resource"=w396) -> ("Numeric"=w394:dbl, "Arduino Resource 2"=w395:T3)  [unwired: 7 in, 1 out]
                }
                frame "9" {
                  n421 = call "sub9choice.vi"("Detector Start Pin"=w397, "Arduino Resource"=w398) -> ("Ouput"=w399:dbl, "Arduino Resource 2"=w400:T3)  [unwired: 7 in, 1 out]
                }
              }
              n422 = Not Equal To 0?(x=w375) -> (x != 0?=w373:bool)
              n423 = case shown="True" w373 {
                tunnel: w372 -> [w383 w387]
                tunnel: [w383 w386] -> w371
                tunnel: [0 1] -> w370
                tunnel: [FALSE TRUE] -> w367
                frame False {
                }
                frame True {
                  n424 = local read "Timeout (sec)"() -> (w388:dbl)
                  n425 = call "subTimeOut.vi"("Timeout (sec)"=w388, "Arduino Resource"=w387) -> ("Arduino Resource 2"=w386:T3)  [unwired: 9 in]
                }
              }
              n426 = local write "Wrong"(w367) -> ()
              n427 = call <vilib>:"Digital Read Pin.vi"("Arduino Resource"=w371, "Digital I/O Pin (0)"=8) -> ("Arduino Resource"=w380:T3, "Value"=w378:u8)  [unwired: 11 in, 1 out]
              n428 = Not Equal To 0?(x=w378) -> (x != 0?=w368:bool)
              n429 = Or(x=w368, y=w367) -> (x .or. y?=w369:bool)
            }
          }
          frame #6 {
            # "ITI Blinking"
            # "Wait for Pellet Box sig"
            n430 = case shown="False" w401 {
              tunnel: w403 -> [w406 w413]
              tunnel: [w405 w413] -> w402
              frame False {
                n431 = while {
                  tunnel: w406 -> [w412]
                  tunnel: [w411] -> w405
                  stop <- w408 stop-if-true
                  n432 = call <vilib>:"Digital Read Pin.vi"("Arduino Resource"=w412, "Digital I/O Pin (0)"=9) -> ("Arduino Resource"=w411:T3, "Value"=w409:u8)  [unwired: 11 in, 1 out]
                  n433 = Not Equal To 0?(x=w409) -> (x != 0?=w408:bool)
                  n434 = Wait (ms)(milliseconds to wait=u32 100) -> ()  [unwired: 1 out]
                }
              }
              frame True {
              }
            }
          }
          frame #7 {
            w419 = FALSE
            w420 = FALSE
            # "Reaction LED Reset"
            # "Indicator LED Reset"
            n435 = while {
              tunnel: [w429] -> w418
              tunnel: w417 -> [w428]
              shift-right: [w424] -> w414
              shift-left: 0 -> [w422]
              stop <- w425 stop-if-true
              w421 = FALSE
              n436 = local write "Correct"(w421) -> ()
              n437 = local write "Wrong"(w421) -> ()
              n438 = local write "ITI"(w421) -> ()
              n439 = flat-sequence {
                tunnel: w428 -> [w433]
                tunnel: [w434] -> w427
                tunnel: [w431] -> w426
                tunnel: [w430] -> w423
                tunnel: w422 -> [w430]
                tunnel: [w470] -> w429
                tunnel: w427 -> [w471]
                tunnel: w426 -> [w472]
                tunnel: [w469] -> w425
                tunnel: [w468] -> w424
                tunnel: w423 -> [w467]
                frame #0 {
                  n440 = Tick Count (ms)() -> (millisecond timer value=w432:u32)
                  n441 = while {
                    tunnel: [w450] -> w434
                    tunnel: w433 -> [w449]
                    tunnel: w432 -> [w448]
                    tunnel: [w435] -> w431
                    stop <- w437 stop-if-true
                    w453 = 1000
                    n442 = local read "Choice Mode"() -> (w443:string)
                    n443 = local read "Detector Pin"() -> (w442:i32)
                    n444 = Tick Count (ms)() -> (millisecond timer value=w454:u32)
                    n445 = case shown="\"9\"" w443 {
                      tunnel: [w457 w461 w466] -> w450
                      tunnel: w449 -> [w458 w462 w464]
                      tunnel: [w456 w460 w465] -> w444
                      tunnel: w442 -> [w455 w459 w463]
                      frame "1" {
                        n446 = call "sub1choice.vi"("Detector Start Pin"=w455, "Arduino Resource"=w458) -> ("Numeric"=w456:dbl, "Arduino Resource 2"=w457:T3)  [unwired: 7 in, 1 out]
                      }
                      frame "5", Default {
                        n447 = call "sub5choice.vi"("Detector Start Pin"=w459, "Arduino Resource"=w462) -> ("Numeric"=w460:dbl, "Arduino Resource 2"=w461:T3)  [unwired: 7 in, 1 out]
                      }
                      frame "9" {
                        n448 = call "sub9choice.vi"("Detector Start Pin"=w463, "Arduino Resource"=w464) -> ("Ouput"=w465:dbl, "Arduino Resource 2"=w466:T3)  [unwired: 7 in, 1 out]
                      }
                    }
                    n449 = Subtract(x=w454, y=w448) -> (x-y=w452:u32)
                    n450 = Multiply(x=w453, y="ITI (sec)") -> (x*y=w446:dbl)
                    n451 = Divide(x=w452, y=w453) -> (x/y=w447:dbl)
                    n452 = Greater Or Equal?(x=w452, y=w446) -> (x >= y?=w436:bool)
                    n453 = Subtract(x="ITI (sec)", y=w447) -> (x-y=w439:dbl)
                    n454 = Not Equal To 0?(x=w444) -> (x != 0?=w435:bool)
                    n455 = Less Than 0?(x=w439) -> (x < 0?=w440:bool)
                    n456 = Or(x=w436, y=w435) -> (x .or. y?=w437:bool)
                    n457 = local write "Wrong"(w435) -> ()
                    n458 = Select(t=0, s=w440, f=w439) -> (s? t:f=→"ITI Remaining":dbl)
                    "ITI" <- TRUE
                  }
                }
                frame #1 {
                  n459 = case shown="True" w472 {
                    tunnel: w471 -> [w475 w482]
                    tunnel: [w475 w476] -> w470
                    tunnel: [TRUE FALSE] -> w469
                    tunnel: [w473 w479] -> w468
                    tunnel: w467 -> [w473 w478]
                    frame False {
                    }
                    frame True {
                      n460 = local read "Timeout (sec)"() -> (w481:dbl)
                      n461 = call "subTimeOut.vi"("Timeout (sec)"=w481, "Arduino Resource"=w482) -> ("Arduino Resource 2"=w477:T3)  [unwired: 9 in]
                      n462 = Increment(x=w478) -> (x+1=w479:i32)
                      n463 = while {
                        tunnel: w477 -> [w492]
                        tunnel: [w491] -> w476
                        i -> [w483]
                        stop <- w488 stop-if-true
                        n464 = Quotient & Remainder(x=w483, y=2) -> (x-y*floor(x/y)=w485:i32)  [unwired: 1 out]
                        n465 = call <vilib>:"Digital Read Pin.vi"("Arduino Resource"=w492, "Digital I/O Pin (0)"=8) -> ("Arduino Resource"=w491:T3, "Value"=w489:u8)  [unwired: 11 in, 1 out]
                        n466 = Equal To 0?(x=w485) -> (x = 0?=w486:bool)
                        n467 = Not Equal To 0?(x=w489) -> (x != 0?=w488:bool)
                        n468 = local write "ITI"(w486) -> ()
                        n469 = Wait (ms)(milliseconds to wait=u32 100) -> ()  [unwired: 1 out]
                      }
                    }
                  }
                }
              }
            }
            n470 = local write "Hole 1"(w419) -> ()
            n471 = local write "Hole 2"(w419) -> ()
            n472 = local write "Hole 3"(w419) -> ()
            n473 = local write "Hole 4"(w419) -> ()
            n474 = local write "Hole 5"(w419) -> ()
            n475 = local write "Hole  1"(w420) -> ()
            n476 = local write "Hole  2"(w420) -> ()
            n477 = local write "Hole  3"(w420) -> ()
            n478 = local write "Hole  4"(w420) -> ()
            n479 = local write "Hole  5"(w420) -> ()
            n480 = local write "Hole  6"(w420) -> ()
            n481 = local write "Hole  7"(w420) -> ()
            n482 = local write "Hole  8"(w420) -> ()
            n483 = local write "Hole  9"(w420) -> ()
            n484 = local write "Hole 6"(w419) -> ()
            n485 = local write "Hole 7"(w419) -> ()
            n486 = local write "Hole 8"(w419) -> ()
            n487 = local write "Hole 9"(w419) -> ()
          }
        }
        n488 = Add(x=1, y=w217) -> (x+y=w215:i32)
        "Current Trial" <- w215
        n489 = local read "# of total Trial"() -> (w214:i32)
        n490 = Less Or Equal?(x=w215, y=w214) -> (x <= y?=→"Experiment Running":bool)
        n491 = call "subturnOnLedForNSec.vi"("Second"="LED On (sec)", "Pin Number"=w213, "Arduino Resource"=w212) -> ()  [unwired: 8 in, 1 out]
        n492 = local read "Current Trial"() -> (w199:dbl)
        n493 = Boolean To (0,1)(Boolean=w218) -> (0, 1=w204:i16)
        n494 = Increment(x=w199) -> (x+1=w197:dbl)
        n495 = Subtract(x=w197, y=5) -> (x-y=w190:dbl)
        n496 = Greater?(x=w197, y=5) -> (0:w194:bool)
        n497 = Build Array(w197, w206, w205, w204, w182, w176, w175) -> (w202:dbl[])
        n498 = Select(t=w190, s=w194, f=0) -> (s? t:f=w195:dbl)
        n499 = Decrement(x=w197) -> (x-1=w198:dbl)
        n500 = Build Array(w195, 0) -> (w196:dbl[])
        n501 = local write "Correct"(w174) -> ()
        n502 = local write "ITI"(w174) -> ()
        n503 = local write "Wrong"(w174) -> ()
        n504 = call-poly <vilib>:"Write To Spreadsheet File.vi"("transpose? (no:F)"=FALSE, "append to file? (new file:F)"=TRUE, "1D data"=w202, "file path (dialog if empty)"=w207) -> ()  [unwired: 4 in, 1 out]
        n505 = Insert Into Array(array=w201, index (row)=w198, new element=w202) -> (w200:i32[][])  [unwired: 1 in]
        "Array" <- w200
        n506 = property on="Array" class="Arr (strict)"("Index Values"=w196) -> ()  [unwired: 2 in, 2 out]
      }
      n507 = while {
        tunnel: w162 -> [w167]
        stop <- w166 continue-if-true
        n508 = Tick Count (ms)() -> (millisecond timer value=w168:u32)
        n509 = Subtract(x=w168, y=w167) -> (x-y=w169:u32)
        n510 = Divide(x=w169, y=1000) -> (x/y=→"Elapsed Time":dbl)
        n511 = local read "Experiment Running"() -> (w166:bool)
        n512 = Wait (ms)(milliseconds to wait=100) -> ()  [unwired: 1 out]
      }
      n513 = local write "Experiment Running"(w161) -> ()
      n514 = call <vilib>:"Close.vi"("Arduino Resource"=w164) -> ()  [unwired: 14 in, 1 out]
    }
  }
